vi "CLAD last day practice.vi"() -> ()   [LabVIEW 2020]
panel:
  out "Numeric 4":i32
  out "result string":string
  out "replaced substring":string
  in  "string 2":string
  in  "substring (\"\")":string
  in  "offset (0) 2":i32
  in  "length (len. of substring)":i32
  out "offset past match":i32
  out "after substring":string
  out "match substring":string
  out "before substring":string
  in  "offset (0)":i32
  in  "regular expression":string
  in  "string":string
  out "Numeric 3":u8
  in  "Numeric 2":u8
  in  "Numeric":u8
  out "element 3":dbl
  out "element 2":dbl
  out "element":dbl
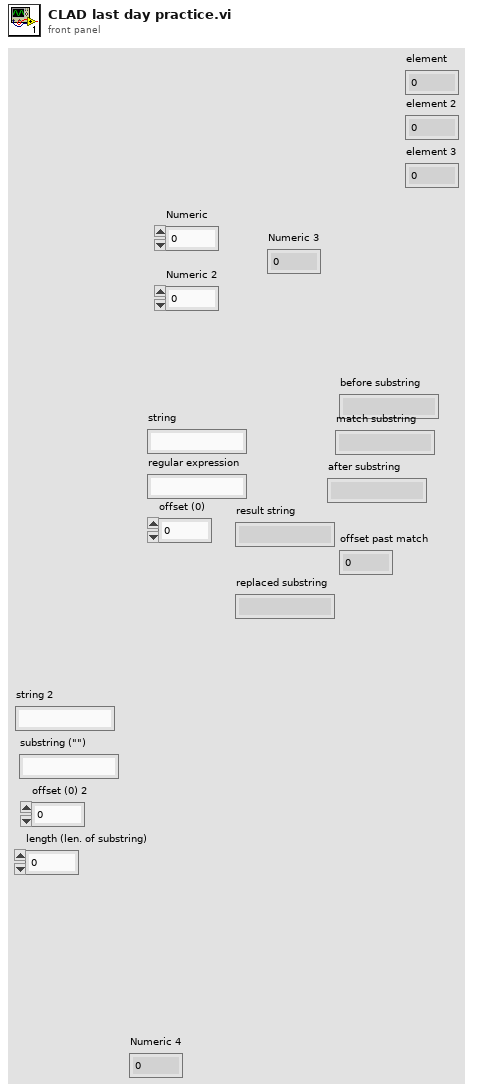
[diagram p1: front panel]
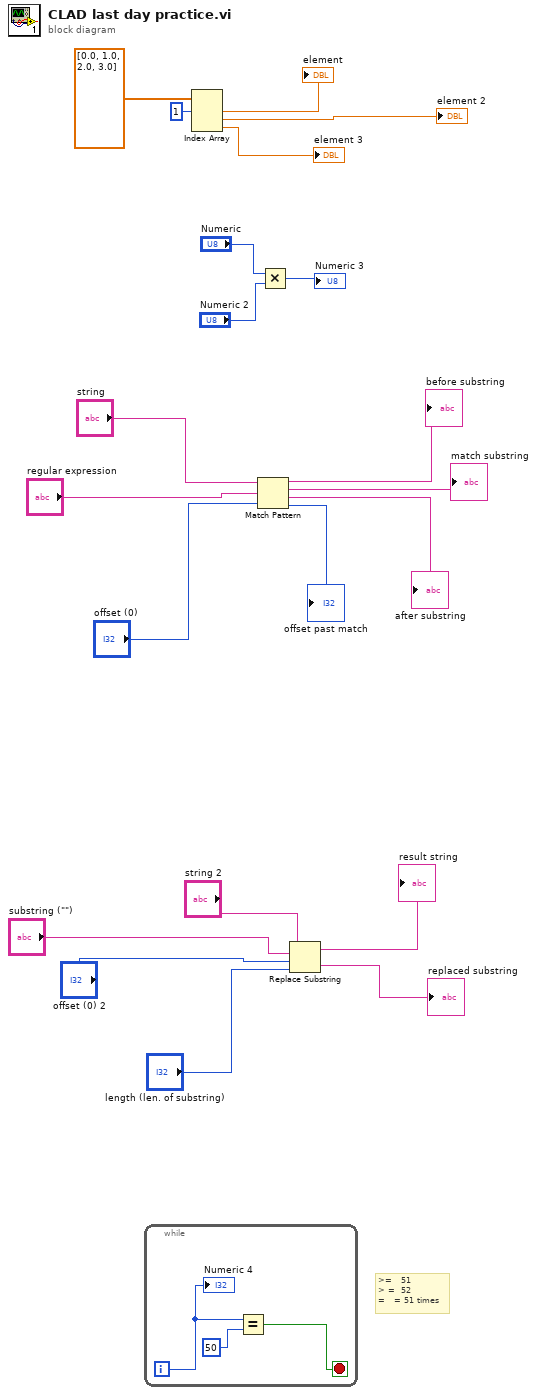
[diagram p0: block diagram]
diagram:
  # ">=   51\n> =  52\n=   = 51 times"
  n1 = while {
    i -> [w22]
    stop <- w23 stop-if-true
    n2 = Equal?(x=w22, y=50) -> (x = y?=w23:bool)
    "Numeric 4" <- w22
  }
  n3 = Index Array "Index Array"(array=dbl[] [0.0, 1.0, 2.0, 3.0], index #1=1 ("index")) -> (element #1=→"element":dbl, element #2=→"element 2":dbl, element #3=→"element 3":dbl)  [unwired: 2 in]
  n4 = Match Pattern(string="string", regular expression="regular expression", offset (0)="offset (0)") -> (before substring=→"before substring":string, match substring=→"match substring":string, after substring=→"after substring":string, offset past match=→"offset past match":i32)
  n5 = Multiply(x="Numeric", y="Numeric 2") -> (x*y=→"Numeric 3":u8)
  n6 = Replace Substring(2:"length (len. of substring)", 3:"offset (0) 2", 4:"substring (\"\")", 5:"string 2") -> (0:→"replaced substring":string, 1:→"result string":string)
